vi "keyboardInput.vi"() -> ()   [LabVIEW 2020]
panel:
  in  "stop 5":bool
  out "Waveform Chart 2":dbl(graph)
  out "text":string
  out "number":dbl
  in  "stop 2":bool
  out "ASCII Char 2":i16
  out "Character 2":string
  out "date string":string
  out "time string":string
  out "standard output 2":string
  out "PID":string
  out "ASCII Char":i16
  out "Character":string
  out "standard output":string
  in  "stop":bool
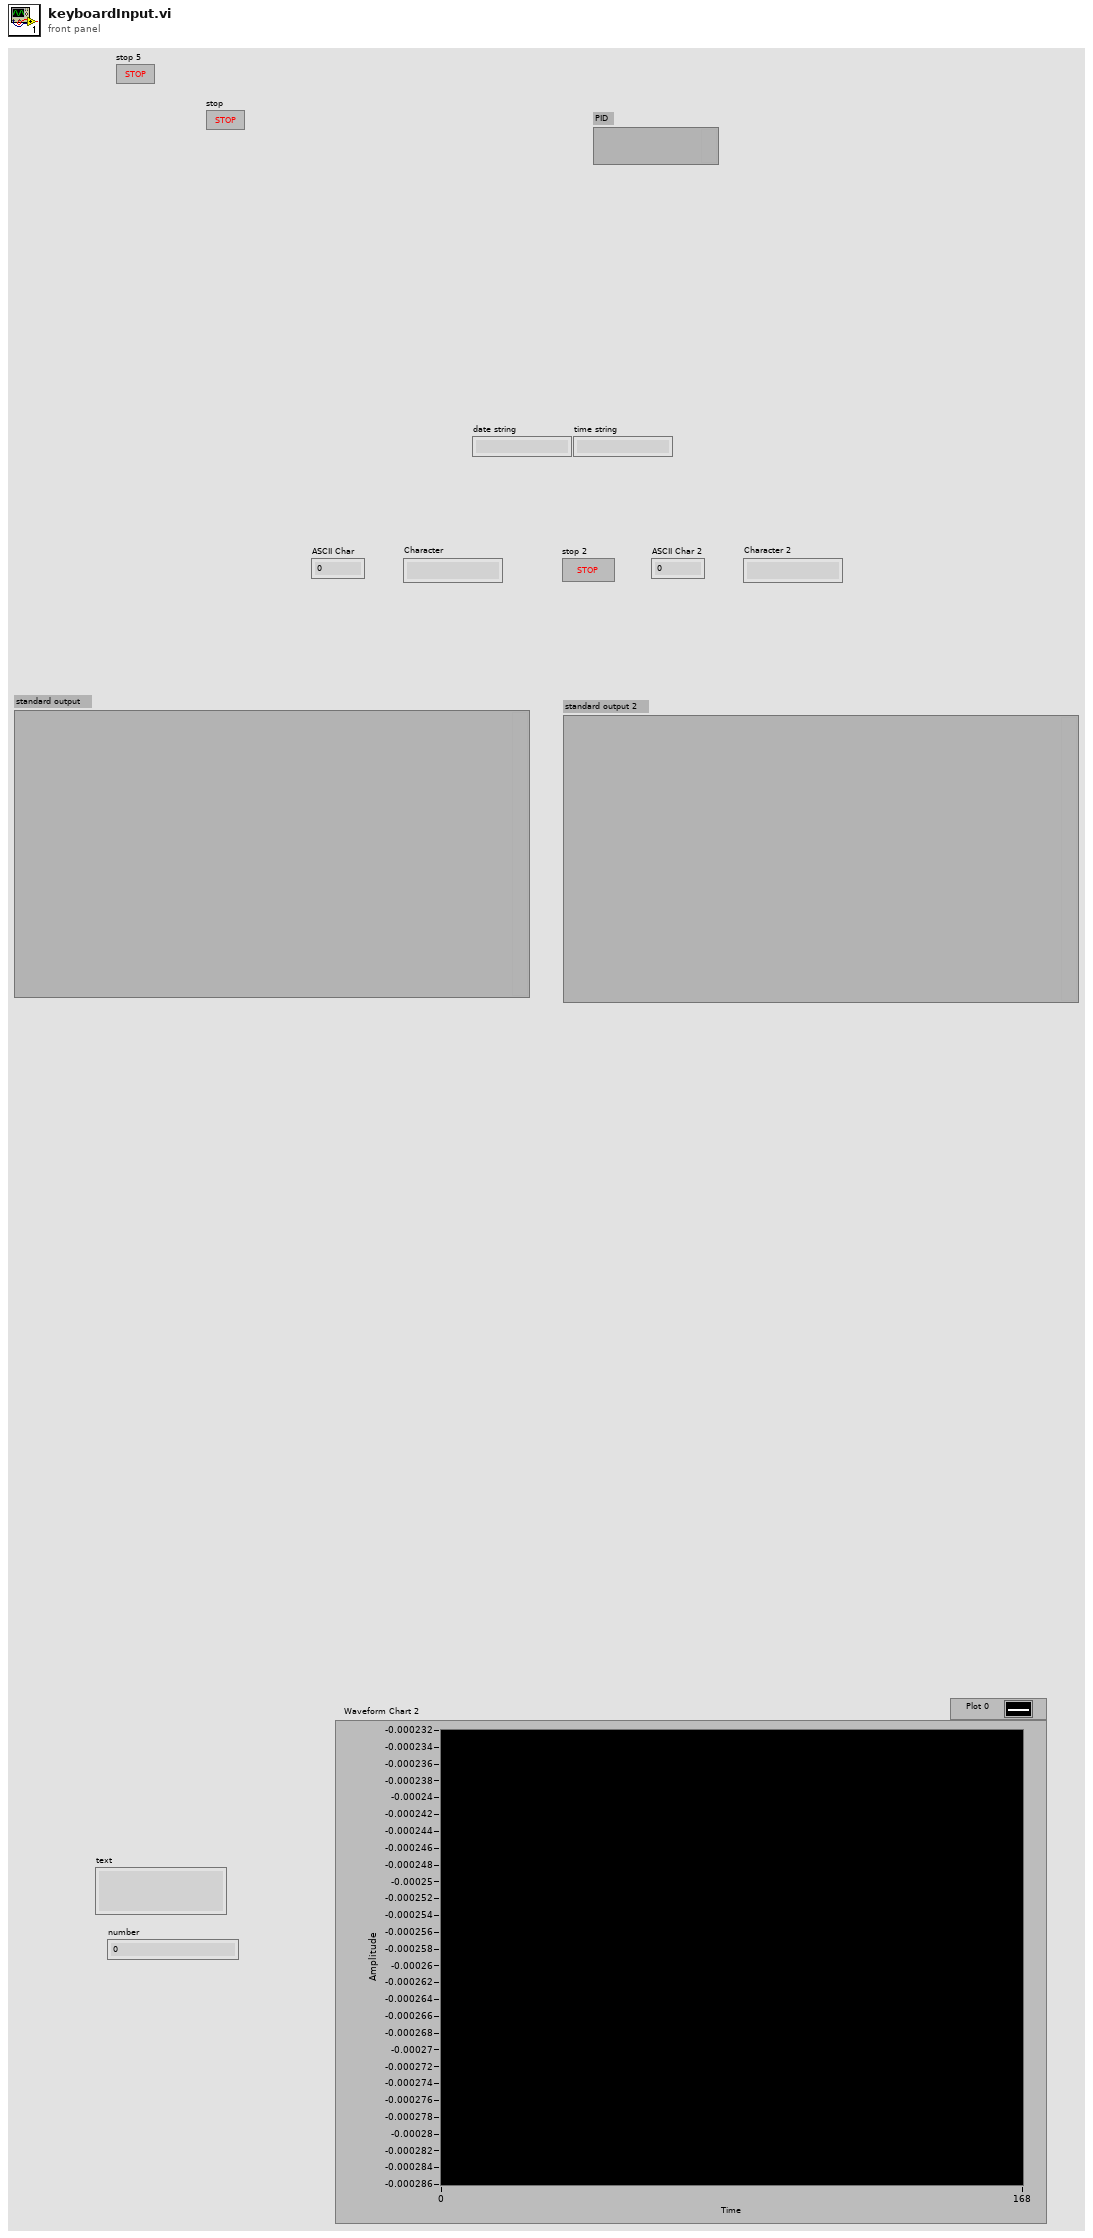
[diagram p1: front panel]
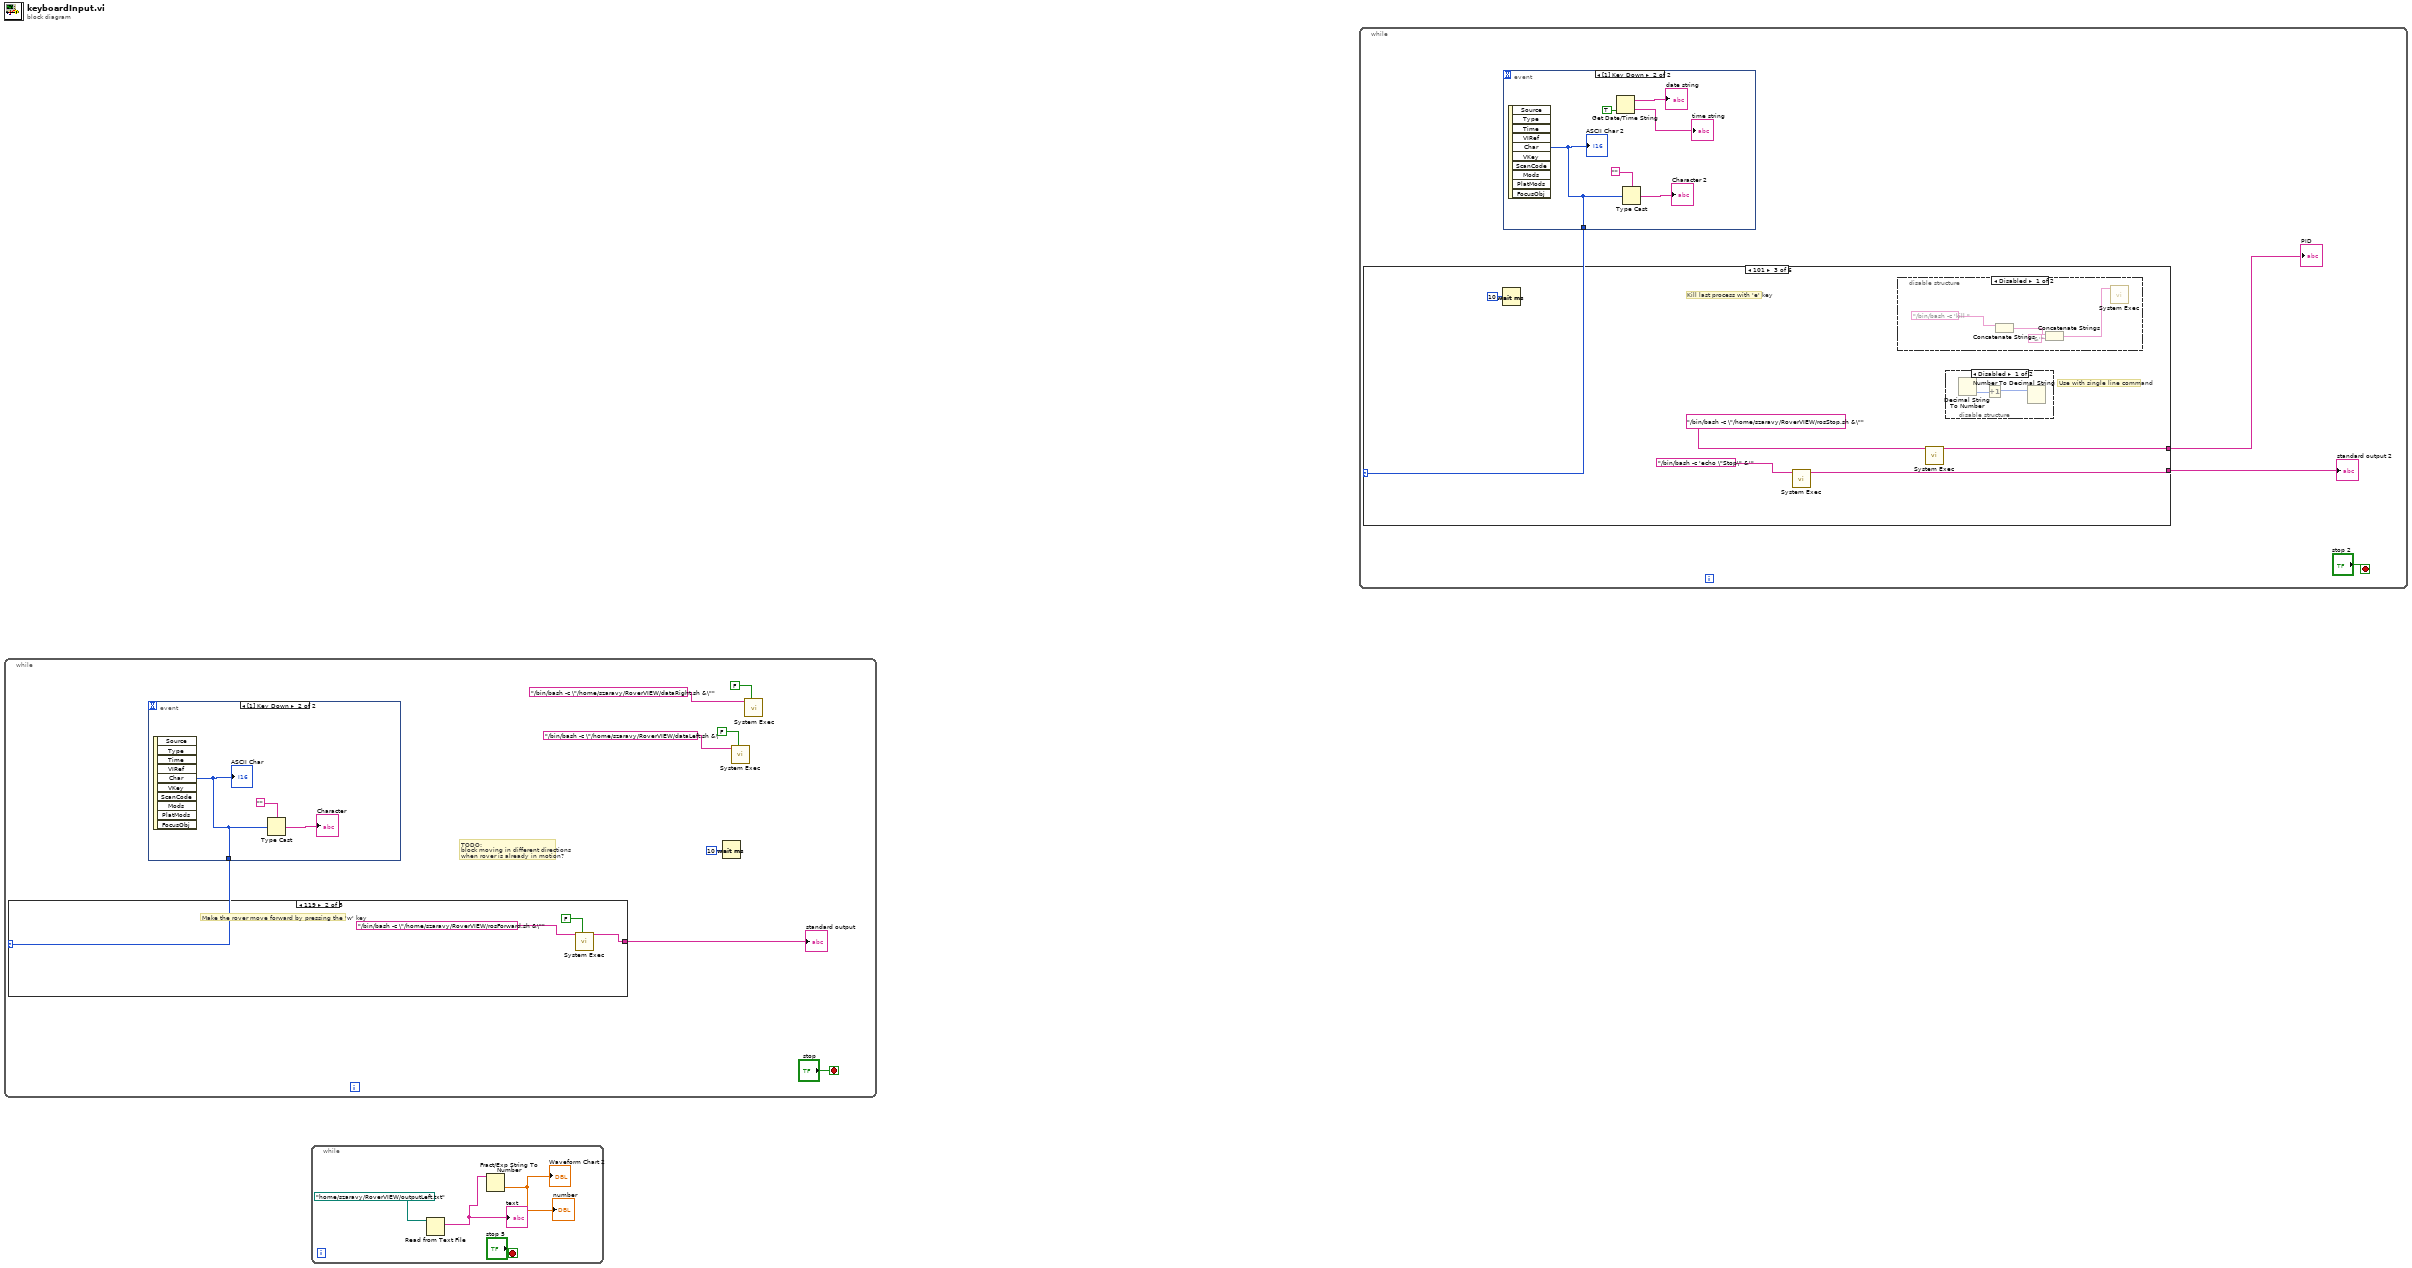
[diagram p0: block diagram]
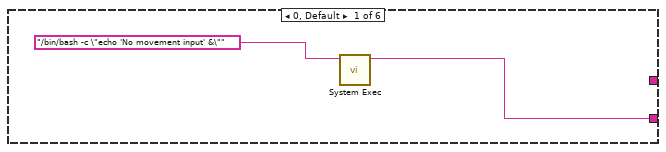
[diagram p2: hidden frame]
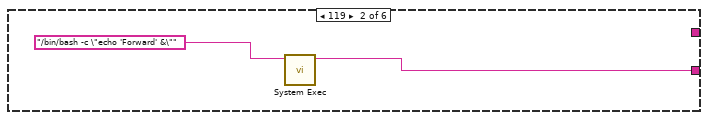
[diagram p3: hidden frame]
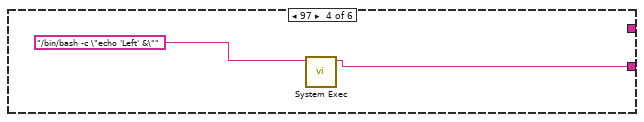
[diagram p6: hidden frame]
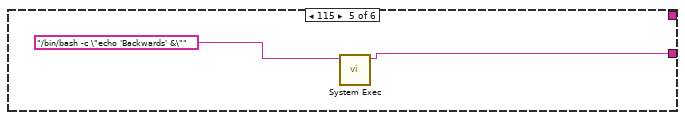
[diagram p7: hidden frame]
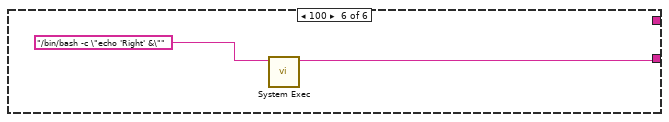
[diagram p8: hidden frame]
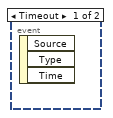
[diagram p9: hidden frame]
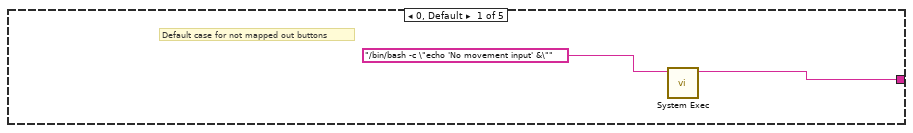
[diagram p10: hidden frame]
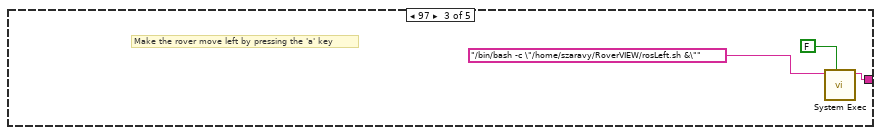
[diagram p11: hidden frame]
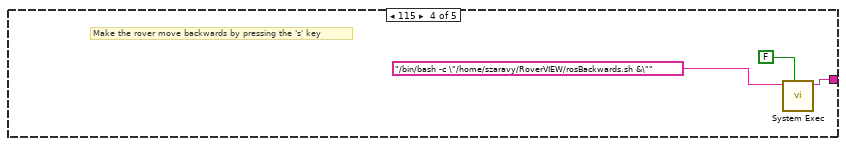
[diagram p12: hidden frame]
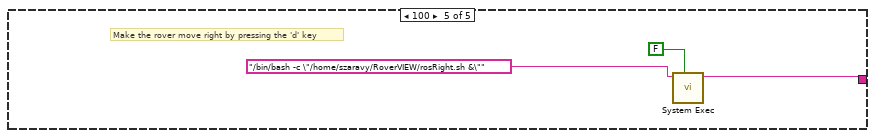
[diagram p13: hidden frame]
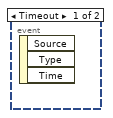
[diagram p14: hidden frame]
diagram:
  n1 = while {
    stop <- "stop" stop-if-true
    # "TODO: \nblock moving in different directions\nwhen rover is already in motion?"
    n2 = event shown="[1] Key Down" {
      selector: _ -> [_ _]
      dyn-events: _ -> [_ _]
      timeout: _ -> [_ _]
      tunnel: [_ w23] -> w8
      event Timeout {
        n3 = event-data() -> ()  [unwired: 1 in, 3 out]
      }
      event Key Down {
        n4 = event-data() -> ("Char"=w23:i16)  [unwired: 1 in, 9 out]
        "ASCII Char" <- w23
        n5 = Type Cast(type="", x=w23) -> (*(type *) &x=→"Character":string)
      }
    }
    n6 = case shown="119" w8 {
      tunnel: [w9 w12 w15 w18 w21] -> w7
      frame 0, Default {
        # "Default case for not mapped out buttons"
        n7 = call <vilib>:"System Exec.vi"("command line"="/bin/bash -c \"echo 'No movement input' &\"") -> ("standard output"=w9:string)  [unwired: 7 in, 3 out]
      }
      frame 119 {
        # "Make the rover move forward by pressing the 'w' key"
        n8 = call <vilib>:"System Exec.vi"("wait until completion? (T)"=FALSE, "command line"="/bin/bash -c \"/home/szaravy/RoverVIEW/rosForward.sh &\"") -> ("standard output"=w12:string)  [unwired: 6 in, 3 out]
      }
      frame 97 {
        # "Make the rover move left by pressing the 'a' key"
        n9 = call <vilib>:"System Exec.vi"("wait until completion? (T)"=FALSE, "command line"="/bin/bash -c \"/home/szaravy/RoverVIEW/rosLeft.sh &\"") -> ("standard output"=w15:string)  [unwired: 6 in, 3 out]
      }
      frame 115 {
        # "Make the rover move backwards by pressing the 's' key"
        n10 = call <vilib>:"System Exec.vi"("wait until completion? (T)"=FALSE, "command line"="/bin/bash -c \"/home/szaravy/RoverVIEW/rosBackwards.sh &\"") -> ("standard output"=w18:string)  [unwired: 6 in, 3 out]
      }
      frame 100 {
        # "Make the rover move right by pressing the 'd' key"
        n11 = call <vilib>:"System Exec.vi"("wait until completion? (T)"=FALSE, "command line"="/bin/bash -c \"/home/szaravy/RoverVIEW/rosRight.sh &\"") -> ("standard output"=w21:string)  [unwired: 6 in, 3 out]
      }
    }
    "standard output" <- w7
    n12 = Wait (ms)(milliseconds to wait=u32 10) -> ()  [unwired: 1 out]
    n13 = call <vilib>:"System Exec.vi"("wait until completion? (T)"=FALSE, "command line"="/bin/bash -c \"/home/szaravy/RoverVIEW/dataLeft.sh &\"") -> ()  [unwired: 6 in, 4 out]
    n14 = call <vilib>:"System Exec.vi"("wait until completion? (T)"=FALSE, "command line"="/bin/bash -c \"/home/szaravy/RoverVIEW/dataRight.sh &\"") -> ()  [unwired: 6 in, 4 out]
  }
  n15 = while {
    stop <- "stop 5" stop-if-true
    n16 = Read from Text File(file (use dialog)=path "/home/szaravy/RoverVIEW/outputLeft.txt") -> (text=w27:string)  [unwired: 3 in, 3 out]
    "text" <- w27
    n17 = Fract/Exp String To Number(string=w27) -> (number=→"Waveform Chart 2" →"number":dbl)  [unwired: 3 in, 1 out]
  }
  n18 = while {
    stop <- "stop 2" stop-if-true
    n19 = event shown="[1] Key Down" {
      selector: _ -> [_ _]
      dyn-events: _ -> [_ _]
      timeout: _ -> [_ _]
      tunnel: [_ w58] -> w32
      event Timeout {
        n20 = event-data() -> ()  [unwired: 1 in, 3 out]
      }
      event Key Down {
        n21 = event-data() -> ("Char"=w58:i16)  [unwired: 1 in, 9 out]
        "ASCII Char 2" <- w58
        n22 = Get Date/Time String(want seconds? (F)=TRUE) -> (date string=→"date string":string, time string=→"time string":string)  [unwired: 2 in]
        n23 = Type Cast(type="", x=w58) -> (*(type *) &x=→"Character 2":string)
      }
    }
    n24 = case shown="101" w32 {
      tunnel: [w34 w36 w41 w49 w51 w53] -> w31
      tunnel: [_ _ w40 _ _ _] -> w30
      frame 0, Default {
        n25 = call <vilib>:"System Exec.vi"("command line"="/bin/bash -c \"echo 'No movement input' &\"") -> ("standard output"=w34:string)  [unwired: 7 in, 3 out]
      }
      frame 119 {
        n26 = call <vilib>:"System Exec.vi"("command line"="/bin/bash -c \"echo 'Forward' &\"") -> ("standard output"=w36:string)  [unwired: 7 in, 3 out]
      }
      frame 101 {
        # "Use with single line command"
        # "Kill last process with 'e' key"
        n27 = Wait (ms)(milliseconds to wait=u32 10) -> ()  [unwired: 1 out]
        n28 = call <vilib>:"System Exec.vi"("command line"="/bin/bash -c 'echo \"Stop\" &'") -> ("standard output"=w41:string)  [unwired: 7 in, 3 out]
        n29 = disable-structure shown="Disabled" {
          frame Disabled {
            n30 = Concatenate Strings("/bin/bash -c 'kill " ("string")) -> (w45:string)  [unwired: 1 in]
            n31 = Concatenate Strings(w45, " &'" ("string")) -> (w43:string)
            n32 = call <vilib>:"System Exec.vi"("command line"=w43) -> ()  [unwired: 7 in, 4 out]
          }
          frame Enabled {
          }
        }
        n33 = call <vilib>:"System Exec.vi"("command line"="/bin/bash -c \"/home/szaravy/RoverVIEW/rosStop.sh &\"") -> ("standard output"=w40:string)  [unwired: 7 in, 3 out]
        n34 = disable-structure shown="Disabled" {
          frame Disabled {
            n35 = Decimal String To Number() -> (number=w47:i32)  [unwired: 3 in, 1 out]
            n36 = Increment(x=w47) -> (x+1=w48:i32)
            n37 = Number To Decimal String(number=w48) -> ()  [unwired: 1 in, 1 out]
          }
          frame Enabled {
          }
        }
      }
      frame 97 {
        n38 = call <vilib>:"System Exec.vi"("command line"="/bin/bash -c \"echo 'Left' &\"") -> ("standard output"=w49:string)  [unwired: 7 in, 3 out]
      }
      frame 115 {
        n39 = call <vilib>:"System Exec.vi"("command line"="/bin/bash -c \"echo 'Backwards' &\"") -> ("standard output"=w51:string)  [unwired: 7 in, 3 out]
      }
      frame 100 {
        n40 = call <vilib>:"System Exec.vi"("command line"="/bin/bash -c \"echo 'Right' &\"") -> ("standard output"=w53:string)  [unwired: 7 in, 3 out]
      }
    }
    "standard output 2" <- w31
    "PID" <- w30
  }
